vi "WPI_CameraBuild CGI.vi"(2 "fps":i32=10, 3 "FPS?":bool, 4 "Get String":string) -> (1 "CGI String":string)   [LabVIEW 2017]
doc: "This software is licensed. Open the labview\\readme\\WPI Robotics Library Open Source License.txt file for more information."
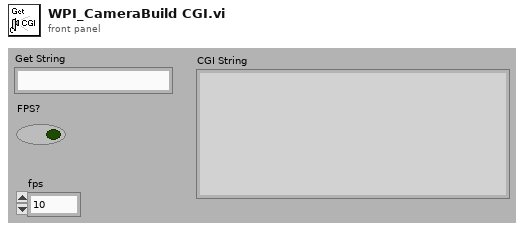
[diagram p1: front panel]
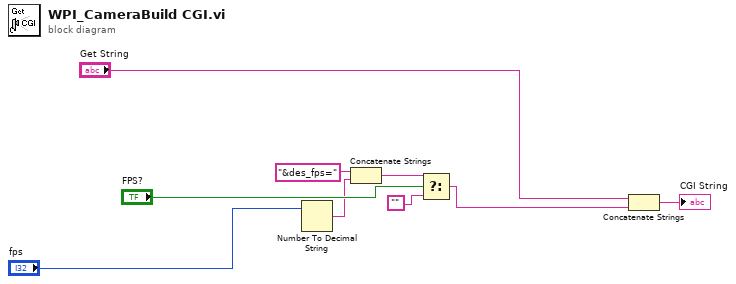
[diagram p0: block diagram]
diagram:
  n1 = Number To Decimal String(number="fps") -> (decimal integer string=w5:string)  [unwired: 1 out]
  n2 = Concatenate Strings("&des_fps=", w5) -> (w4:string)
  n3 = Select(t=w4, s="FPS?", f="") -> (s? t:f=w1:string)
  n4 = Concatenate Strings("Get String", w1) -> (→"CGI String":string)
